vi "RSZVB Get Limit Check.vi"(8 "error in (no error)":errorcluster {"code" format="%.0x"}, 9 "Limit Line (3: All)":i32(ring)=3 items=["Upper"=1, "Lower"=2, "All"=3], 10 "Channel (Trace) (1)":i32=1, 11 "VISA session":refnum<visa-resource-name>) -> (0 "error out":errorcluster {"code" format="%.0x"}, 2 "Limit Check":bool, 3 "dup VISA session":refnum<visa-resource-name>)   [LabVIEW 2011]
doc: "This VI returns if the limit check (or individual upper and lower limits) is switched on or off.\n\nRemote-control command(s):\nCALCulate<Ch/Tr>:LIMit:STATe?\nCALCulate<Ch/Tr>:LIMit:LOWer:STATe?\nCALCulate<Ch/Tr>:LIMit:UPPer:STATe?"
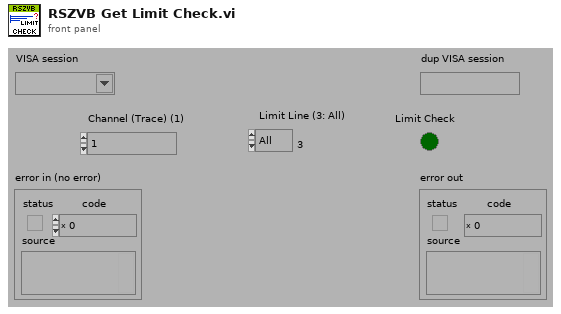
[diagram p1: front panel]
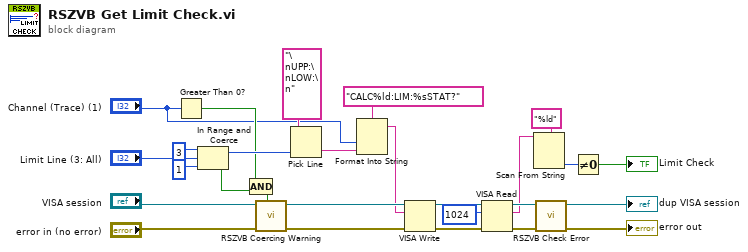
[diagram p0: block diagram]
diagram:
  n1 = Greater Than 0?(x="Channel (Trace) (1)") -> (x > 0?=w17:bool)
  n2 = In Range and Coerce(upper limit=3, x="Limit Line (3: All)", lower limit=1) -> (coerced(x)=w24:i32, In Range?=w18:bool)
  n3 = Compound Arithmetic op=AND(w17, w18) -> (w16:bool)
  n4 = call "RSZVB Coercing Warning.vi"("In Range?"=w16, "error in (no error)"="error in (no error)", "VISA session"="VISA session") -> ("error out"=w21:errorcluster, "dup VISA session"=w22:refnum<visa-resource-name>)  [unwired: 7 in]
  n5 = Pick Line(multi-line string="\nUPP:\nLOW:\n", line index=w24) -> (output string=w19:string)  [unwired: 1 in]
  n6 = Format Into String(format string="CALC%ld:LIM:%sSTAT?", "Channel (Trace) (1)", w19) -> (resulting string=w15:string)  [unwired: 2 in, 1 out]
  n7 = VISA Write(VISA resource name=w22, write buffer=w15, error in (no error)=w21) -> (VISA resource name out=w20:refnum<visa-resource-name>, error out=w4:errorcluster)  [unwired: 1 out]
  n8 = VISA Read(VISA resource name=w20, byte count=u32 1024 ("byte count (0)"), error in (no error)=w4) -> (VISA resource name out=w9:refnum<visa-resource-name>, read buffer=w6:string, error out=w8:errorcluster)  [unwired: 1 out]
  n9 = Scan From String(format string="%ld", input string=w6) -> (output 1=w5:i32)  [unwired: 3 in, 3 out]
  n10 = call "RSZVB Check Error.vi"("error in (no error)"=w8, "VISA session"=w9) -> ("error out"=→"error out":errorcluster, "dup VISA session"=→"dup VISA session":refnum<visa-resource-name>)  [unwired: 8 in]
  n11 = Not Equal To 0?(x=w5) -> (x != 0?=→"Limit Check":bool)
